vi "Event Messenger Channel Lesson 1.vi"() -> ()   [LabVIEW 2019]
doc: "Lesson 1 shows a 1-to-1 example of a channel writer connecting to an Event structure using an Event Messenger channel wire."
uses:
  <extravilib>/ChannelInstances/Event Messenger-i32/Instantiate.vi
  <extravilib>/ChannelInstances/Event Messenger-i32/))Channel.vi
  <extravilib>/ChannelInstances/Event Messenger-i32.lvlib
panel:
  out "Producer":i32
  out "Aborted?":bool
  out "Number of times clicked":i32
  in  "Click Me":bool
  out "Consumer":i32
  in  "Abort":bool
  in  "Stop":bool
  # "Overview: This VI demonstrates how to use the Event Messenger channel wire.\n\nAn Event Messenger channel is a forkable channel that allows you to connect one or more data sources to one or more Event structures. Every time a writer endpoint puts data into the channel, an event will fire, and a waiting Event structure will be able to read the data. \n\nThis first lesson shows a basic 1-to-1 use case. Later lessons demonstrate more complex communication scenarios.\n\n\nInstructions:\n1. Run the VI. Notice that the Producer runs faster than the Consumer. \n2. While the VI is running, press the Click Me button. Each time you do, the counter will be incremented.\n3. Stop the VI in one of two ways:\nIf you hit the Stop button, the Consumer will continue running until the channel is empty of data.\nIf you hit the Abort button, the Consumer will stop immediately.\n4. Open the block diagram. Review the comments there to see how this VI works."
  # "See explanation on block diagram for why clicks on this button are handled slowly."
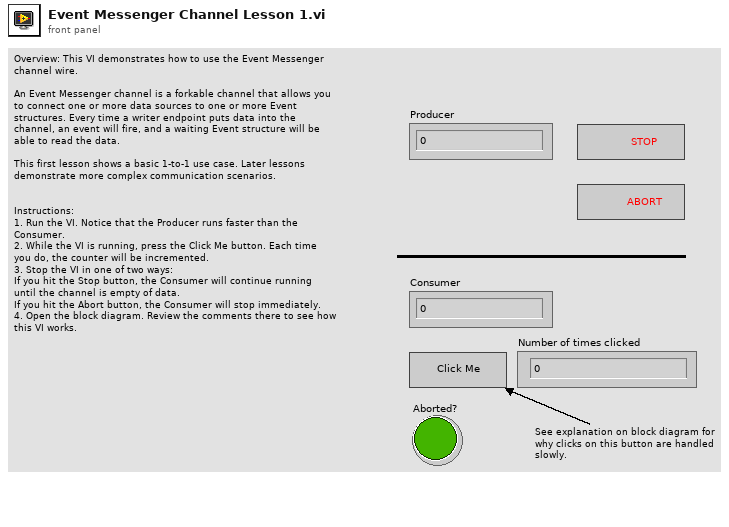
[diagram p1: front panel]
types:
  T1 = typedef "Event Messenger-i32.lvlib/))Channel.ctl" = refnum<queue>
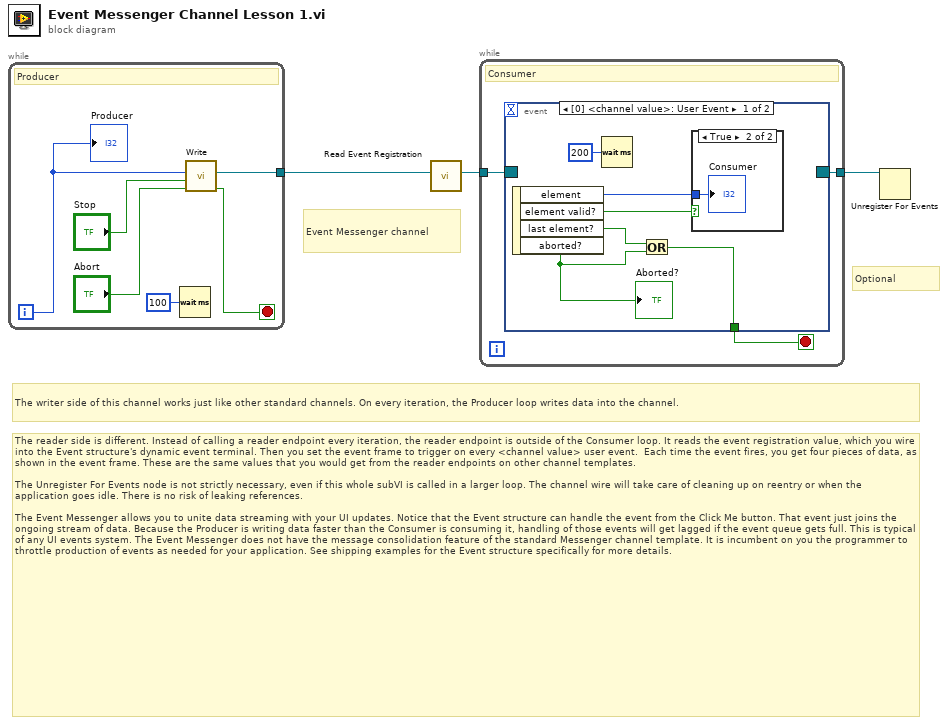
[diagram p0: block diagram]
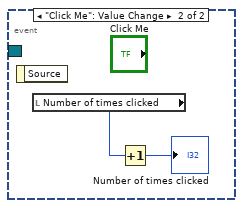
[diagram p3: hidden frame]
diagram:
  # "Optional"
  # "Event Messenger channel"
  # "The reader side is different. Instead of calling a reader endpoint every iteration, the reader endpoint is outside of the Consumer loop. It reads the event registration value, which you wire into the Event structure's dynamic event terminal. Then you set the event frame to trigger on every <channel value> user event.  Each time the event fires, you get four pieces of data, as shown in the event frame. These are the same values that you would get from the reader endpoints on other channel templates.\n\nThe Unregister For Events node is not strictly necessary, even if this whole subVI is called in a larger loop. The channel wire will take care of cleaning up on reentry or when the application goes idle. There is no risk of leaking references.\n\nThe Event Messenger allows you to unite data streaming with your UI updates. Notice that the Event structure can handle the event from the Click Me button. That event just joins the ongoing stream of data. Because the Producer is writing data faster than the Consumer is consuming it, handling of those events will get lagged if the event queue gets full. This is typical of any UI events system. The Event Messenger does not have the message consolidation feature of the standard Messenger channel template. It is incumbent on you the programmer to throttle production of events as needed for your application. See shipping examples for the Event structure specifically for more details."
  # "The writer side of this channel works just like other standard channels. On every iteration, the Producer loop writes data into the channel."
  n1 = while {
    tunnel: [w5] -> w3
    i -> [w9]
    stop <- w7 stop-if-true
    # "Producer"
    n2 = Wait (ms)(milliseconds to wait=u32 100) -> ()  [unwired: 1 out]
    n3 = call <extravilib>:"Write.vi"("abort (F)"="Abort", "last element? (F)"="Stop", "element"=w9) -> ("done?"=w7:bool, "channel"=w5:T1)  [unwired: 7 in]
    "Producer" <- w9
  }
  n4 = call <extravilib>:"Read Event Registration.vi"("channel"=w3) -> ("event registration refnum"=w2:refnum<event-registration>)  [unwired: 10 in]
  n5 = while {
    tunnel: w2 -> [w12]
    tunnel: [w10] -> w1
    stop <- w11 stop-if-true
    # "Consumer"
    n6 = event shown="[0] <channel value>: User Event" {
      selector: w12 -> [_ _]
      dyn-events: [_ _] -> w10
      timeout: _ -> [_ _]
      tunnel: [w13 _] -> w11
      event User Event {
        n7 = event-data() -> ("element"=w18:i32, "element valid?"=w17:bool, "last element?"=w15:bool, "aborted?"=w14:bool)  [unwired: 1 in]
        "Aborted?" <- w14
        n8 = Wait (ms)(milliseconds to wait=u32 200) -> ()  [unwired: 1 out]
        n9 = Or(x=w15, y=w14) -> (x .or. y?=w13:bool)
        n10 = case shown="True" w17 {
          tunnel: w18 -> [_ w19]
          frame False {
          }
          frame True {
            "Consumer" <- w19
          }
        }
      }
      event "Click Me": Value Change {
        n11 = event-data() -> ()  [unwired: 1 in, 1 out]
        n12 = local read "Number of times clicked"() -> (w20:i32)
        n13 = Increment(x=w20) -> (x+1=→"Number of times clicked":i32)
      }
    }
  }
  n14 = Unregister For Events(event registration refnum=w1) -> ()  [unwired: 1 in, 1 out]
